vi "IMAQdx Extract Image.vi"(5 "Timeout (ms)":i32=5000, 6 "Release Previous (true)":bool=TRUE, 7 "Buffer Number Mode (Next)":T1, 8 "error in":errorcluster, 9 "Buffer Number In":u32, 11 "Session In":T3) -> (0 "error out":errorcluster, 1 "Buffer Number Out":u32, 2 "Image Out":T2, 3 "Session Out":T3)   [LabVIEW 2020, in "NI_Vision_Acquisition_Software.lvlib"]
doc: "Retrieves an acquired image directly from the circular buffer list, and does not make a copy of the image. This function is valid only within the context of a ring acquisition."
uses:
  NI_Vision_Acquisition_Software.lvlib
  IMAQdx.ctl
  IMAQ Image.ctl
  IMAQdx Buffer Number Mode.ctl
  niimaqdx.dll
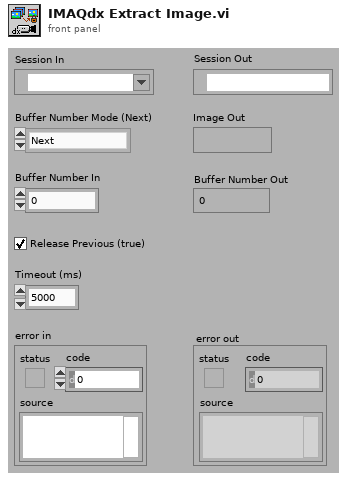
[diagram p1: front panel]
types:
  T1 = typedef "NI_Vision_Acquisition_Software.lvlib/IMAQdx Buffer Number Mode.ctl" = enum32{"Next", "Last", "Buffer Number", "Every", "Last New"}
  T2 = typedef "IMAQ Image.ctl" = refnum<image>
  T3 = typedef "IMAQdx.ctl" = refnum<k21>
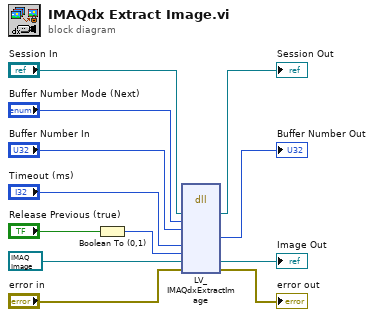
[diagram p0: block diagram]
diagram:
  n1 = Boolean To (0,1)(Boolean="Release Previous (true)") -> (0, 1=w2:i16)
  n2 = dll-call lib="niimaqdx.dll" fn="LV_IMAQdxExtractImage"("refnum"="Session In", "mode"="Buffer Number Mode (Next)", "bufferNumberDesired"="Buffer Number In", "timeoutMs"="Timeout (ms)", "releasePrevious"=w2, "image"=T2 refnum ("Image Out"), "error"="error in") -> ("refnum"=→"Session Out":T3, "bufferNumberActual"=→"Buffer Number Out":u32, "image"=→"Image Out":T2, "error"=→"error out":errorcluster)  [unwired: 9 in, 2 out]
